vi "sequence.vi"() -> ()   [LabVIEW 2021]
panel:
  out "Array":string[](array[string])
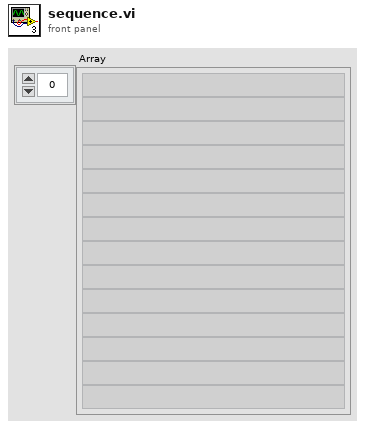
[diagram p1: front panel]
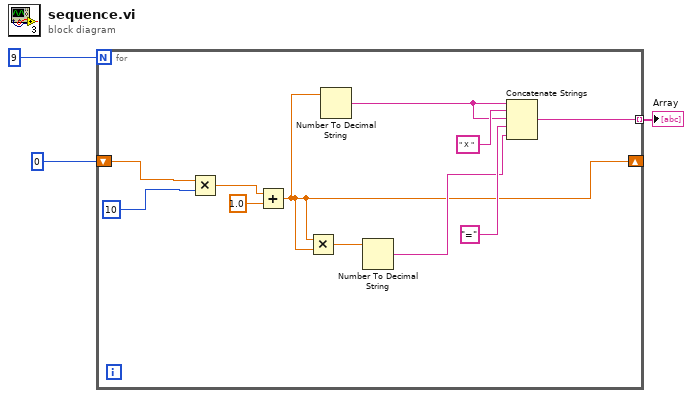
[diagram p0: block diagram]
diagram:
  n1 = for {
    N: 9 -> [_]
    shift-right: [w4] -> _
    shift-left: 0 -> [w14]
    tunnel: [w5] -> w1 mode=indexing
    n2 = Multiply(x=w14, y=10) -> (x*y=w11:dbl)
    n3 = Add(x=w11, y=1.0) -> (x+y=w4:dbl)
    n4 = Multiply(x=w4, y=w4) -> (x*y=w7:dbl)
    n5 = Number To Decimal String(number=w4) -> (decimal integer string=w9:string)  [unwired: 1 in]
    n6 = Number To Decimal String(number=w7) -> (decimal integer string=w6:string)  [unwired: 1 in]
    n7 = Concatenate Strings(w9, " X ", w9, "=", w6) -> (w5:string)
  }
  "Array" <- w1
